vi "Simulation Time Elapsed.vi"(8 "error in (no error)":errorcluster, 10 "Time Target (s)":sgl, 11 "first step?":bool) -> (0 "error out":errorcluster, 3 "Time Elapsed?":bool, 4 "Time":sgl)   [LabVIEW 2013]
uses:
  <vilib>/robotics/Simulator/Interface/Simulator References/Get World Reference.vi
  <vilib>/robotics/Simulator/NI_Robotics_Simulator.lvlib
  <resource>/objmgr/LVODE.rc
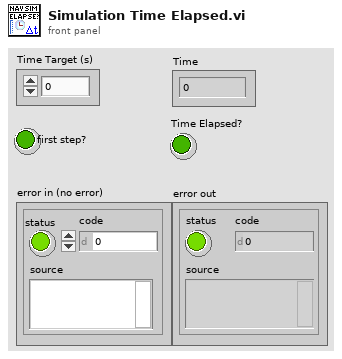
[diagram p1: front panel]
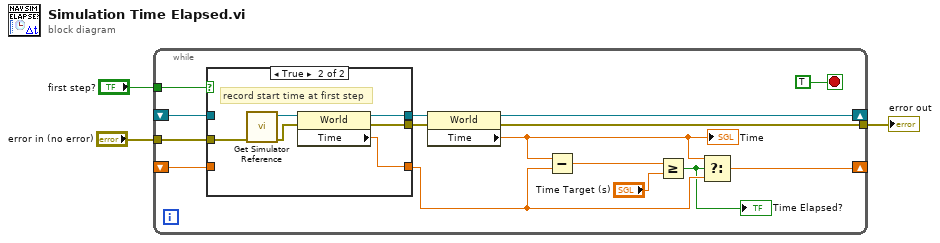
[diagram p0: block diagram]
diagram:
  n1 = while {
    tunnel: "error in (no error)" -> [w18]
    tunnel: [w12] -> w2
    shift-right: [w13] -> _
    shift-left: _ -> [w17]
    shift-right: [w9] -> _
    shift-left: _ -> [w16]
    tunnel: "first step?" -> [w5]
    stop <- TRUE stop-if-true
    n2 = case shown="True" w5 {
      tunnel: [w19 w25] -> w14
      tunnel: w18 -> [w19 w24]
      tunnel: [w21 w23] -> w15
      tunnel: w17 -> [w21 _]
      tunnel: [w20 w22] -> w8
      tunnel: w16 -> [w20 _]
      frame False {
      }
      frame True {
        # "record start time at first step"
        n3 = call-poly <vilib>:"Get Simulator Reference.vi"("error in (no error)"=w24) -> ("error out"=w26:errorcluster, "world ref"=w27:refnum<k20>)  [unwired: 9 in]
        n4 = property class="World"(reference=w27, error in=w26) -> (reference out=w23:refnum<k20>, error out=w25:errorcluster, "Time"=w22:sgl)
      }
    }
    n5 = property class="World"(reference=w15, error in=w14) -> (reference out=w13:refnum<k20>, error out=w12:errorcluster, "Time"=w6:sgl)
    "Time" <- w6
    n6 = Subtract(x=w6, y=w8) -> (x-y=w7:sgl)
    n7 = Greater Or Equal?(x=w7, y="Time Target (s)") -> (x >= y?=w4:bool)
    "Time Elapsed?" <- w4
    n8 = Select(t=w6, s=w4, f=w8) -> (s? t:f=w9:sgl)
  }
  "error out" <- w2
